vi "EuniceF_Project3LABVIEW.vi"() -> ()   [LabVIEW 2025]
panel:
  out "Low Level":bool
  out "Flow Rate, L/s":dbl(slide) scale=0.0..7.0 scale format="%1_3f"
  out "Head, m":dbl(slide) scale=0.0..2.5 scale format="%1_3f"
  out "Level, m":dbl(slide) scale=0.0..6.0 scale format="%#_2f"
  out "Pressure, kPa":dbl(slide) scale=0.0..65.0 scale format="%2_3f"
  out "I,mA":dbl(slide) scale=0.0..22.0 scale format="%2_3f"
  out "Vfrom,I":dbl(slide) scale=-5.0..-1.0 scale format="%3.2f"
  out "Vscc,V":dbl(slide) scale=-5.0..5.0 scale format="%3.2f"
  out "AtoD":i16
  in  "stop":bool
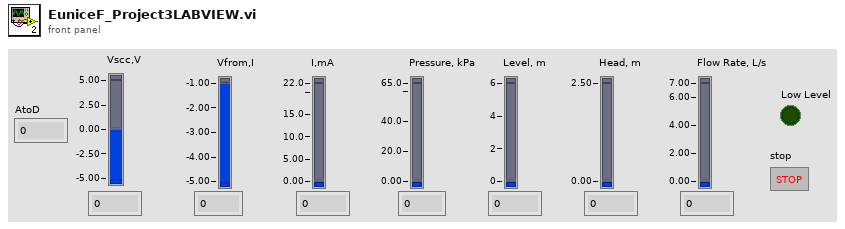
[diagram p1: front panel]
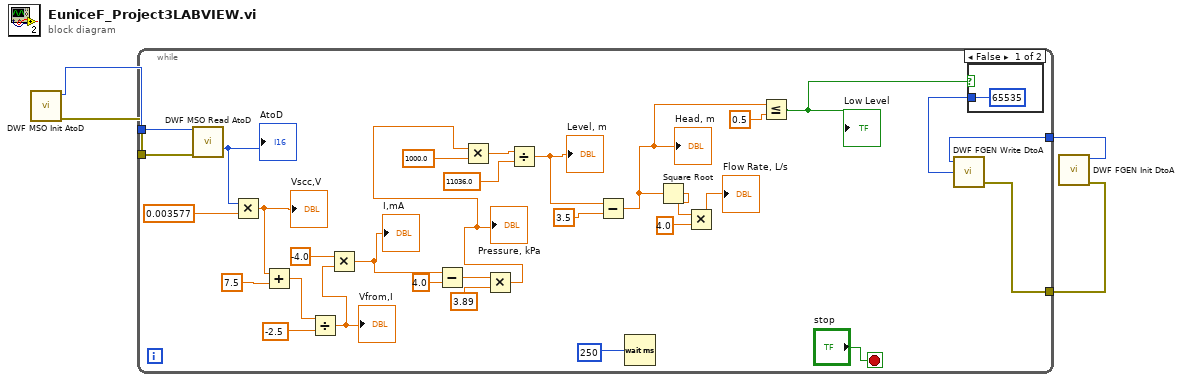
[diagram p0: block diagram]
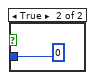
[diagram p2: hidden frame]
diagram:
  n1 = call "DWF MSO Init AtoD.vi"() -> ("Error Out"=w3:errorcluster, "Instrument Handle Out"=w4:i32)  [unwired: 10 in]
  n2 = call "DWF FGEN Init DtoA.vi"() -> ("Error Out"=w2:errorcluster, "Instrument Handle Out"=w1:u32)  [unwired: 10 in]
  n3 = while {
    tunnel: w4 -> [w35]
    tunnel: w3 -> [w34]
    tunnel: w2 -> [w9]
    tunnel: w1 -> [w8]
    stop <- "stop" stop-if-true
    n4 = call "DWF MSO Read AtoD.vi"("Instrument Handle In AtoD"=w35, "Error In"=w34) -> ("AtoD"=w32:i16)  [unwired: 12 in, 1 out]
    "AtoD" <- w32
    n5 = Multiply(x=w32, y=0.003577) -> (x*y=w30:dbl)
    "Vscc,V" <- w30
    n6 = Add(x=w30, y=7.5) -> (x+y=w28:dbl)
    n7 = Divide(x=w28, y=-2.5) -> (x/y=w26:dbl)
    "Vfrom,I" <- w26
    n8 = Multiply(x=-4.0, y=w26) -> (x*y=w25:dbl)
    "I,mA" <- w25
    n9 = Subtract(x=w25, y=4.0) -> (x-y=w23:dbl)
    n10 = Multiply(x=w23, y=3.89) -> (x*y=w20:dbl)
    "Pressure, kPa" <- w20
    n11 = Multiply(x=w20, y=1000.0) -> (x*y=w19:dbl)
    n12 = Divide(x=w19, y=11036.0) -> (x/y=w16:dbl)
    "Level, m" <- w16
    n13 = Subtract(x=w16, y=3.5) -> (x-y=w10:dbl)
    "Head, m" <- w10
    n14 = Wait (ms)(milliseconds to wait=u32 250) -> ()  [unwired: 1 out]
    n15 = Square Root(x=w10) -> (sqrt(x)=w13:dbl)
    n16 = Multiply(x=w13, y=4.0) -> (x*y=→"Flow Rate, L/s":dbl)
    n17 = Less Or Equal?(x=w10, y=0.5) -> (x <= y?=w7:bool)
    "Low Level" <- w7
    n18 = case shown="False" w7 {
      tunnel: [65535 0] -> w6
      frame False {
      }
      frame True {
      }
    }
    n19 = call "DWF FGEN Write DtoA.vi"("Error In"=w9, "Raw Data"=w6, "Instrument Handle In"=w8) -> ()  [unwired: 1 in, 2 out]
  }
